vi "read_data.vi"(8 "error in (no error)":errorcluster, 11 "IsotonicRegression in":refnum<class "IsotonicRegression.lvclass">) -> (0 "error out":errorcluster, 2 "data":T1, 3 "IsotonicRegression out":refnum<class "IsotonicRegression.lvclass">)   [LabVIEW 2020, in "IsotonicRegression.lvclass"]
uses:
  IsotonicRegression.lvclass
  Controls/isotonic_regression_data.ctl
  IsotonicRegression.lvclass/IsotonicRegression.ctl
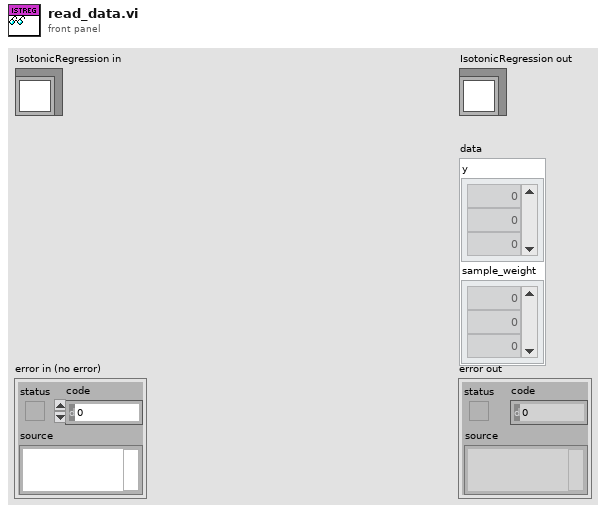
[diagram p1: front panel]
types:
  T1 = typedef "isotonic_regression_data.ctl" = cluster{"y":dbl[], "sample_weight":dbl[]}
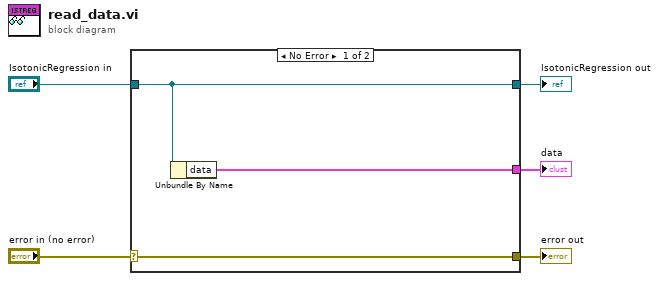
[diagram p0: block diagram]
diagram:
  n1 = case shown="No Error" "error in (no error)" {
    selector: "error in (no error)" -> [w8 w9]
    tunnel: [w8 w9] -> w4
    tunnel: [w7 w10] -> w2
    tunnel: "IsotonicRegression in" -> [w7 w10]
    tunnel: [w6 _] -> w1
    frame No Error {
      n2 = Unbundle By Name(w7) -> ("data"=w6:T1)
    }
    frame Error {
    }
  }
  "error out" <- w4
  "IsotonicRegression out" <- w2
  "data" <- w1
